vi "processPubDataSubscribe.vi"(8 "error in (no error)":errorcluster, 11 "MiddlewareSALThisComponent in":refnum<class "MiddlewareSALThisComponent.lvclass">) -> (0 "error out":errorcluster, 3 "MiddlewareSALThisComponent out":refnum<class "MiddlewareSALThisComponent.lvclass">)   [LabVIEW 2016, in "MiddlewareSALThisComponent.lvclass"]
uses:
  MiddlewareSALThisComponent.lvclass
  home/harini/tcs/ts_sedspectrometer/ComponentTemplateCore/ComponentModel/ComponentModel/Middleware/Middleware.lvclass
  ComponentTemplateCore/ComponentModel/ComponentModel/Middleware/Middleware.lvclass/Middleware.ctl
  ComponentTemplateCore/ComponentModel/ComponentModel/MiddlewareProcessEvent/MiddlewareProcessEvent.lvclass/MiddlewareProcessEvent.ctl
  PubSubDataEvent/PubSubDataEvent.lvclass/PubSubDataEvent.ctl
  ComponentTemplateCore/ComponentModel/ComponentModel/Middleware/Middleware.lvclass
  ComponentTemplateCore/ComponentModel/ComponentModel/MiddlewareProcessEvent/MiddlewareProcessEvent.lvclass
  PubSubDataEvent/PubSubDataEvent.lvclass
  ProgrammaticInitialization/ProgrammaticInitialization.lvclass
  ts_sallv_sedspectrometer/SALLV_calibrationSpectrometer.lvlib
panel:
  out "stopIsTrue":bool
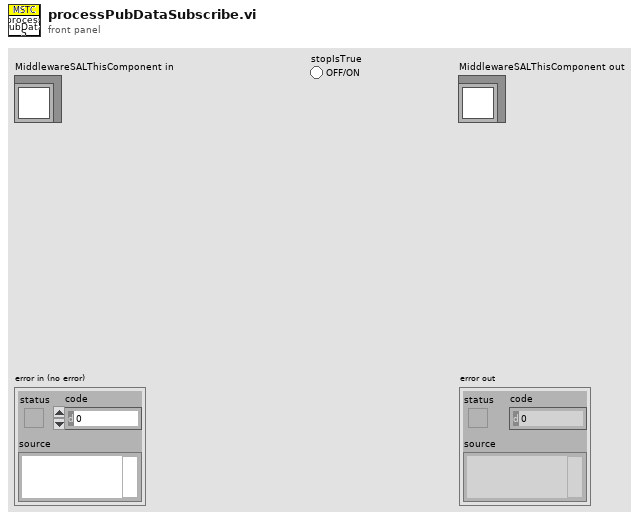
[diagram p1: front panel]
types:
  T1 = typedef "MiddlewareProcessEvents.ctl" = cluster{"disconnect":refnum<user-event>, "error":refnum<user-event>}
  T2 = cluster{"Event Registration Refnum":refnum<event-registration>, "Event Registration Refnum":refnum<event-registration>}
  T3 = typedef "TypedefsDataEvents.lvlib/PubDataEvents.ctl" = cluster{"AppliedSettingsMatchStart":refnum<user-event>, "SettingVersions":refnum<user-event>, "SummaryState":refnum<user-event>, "RejectedCommand":refnum<user-event>, "DetailedState":refnum<user-event>, "ErrorCode":refnum<user-event>, "Heartbeat":refnum<user-event>, "LoopTime_ms":refnum<user-event>, "LoopTimeOutOfRange":refnum<user-event>, "Timestamp":refnum<user-event>, "TimeOut":refnum<user-event>, "MeasuredSpectrum":refnum<user-event>}
  T4 = typedef "SALLV_calibrationSpectrometer.lvlib/logevent_DetailedState.ctl" = cluster{"detailedState":enum16{"", "DisabledState", "EnabledState", "FaultState", "OfflineState", "StandbyState"}, "priority":i32}
  T5 = typedef "SALLV_calibrationSpectrometer.lvlib/logevent_ErrorCode.ctl" = cluster{"errorCode":i32, "priority":i32}
  T6 = typedef "SALLV_calibrationSpectrometer.lvlib/logevent_Heartbeat.ctl" = cluster{"heartbeat":bool, "priority":i32}
  T7 = typedef "SALLV_calibrationSpectrometer.lvlib/LoopTime_ms.ctl" = cluster{"loopTime_ms":dbl}
  T8 = typedef "SALLV_calibrationSpectrometer.lvlib/logevent_LoopTimeOutOfRange.ctl" = cluster{"loopTimeOutOfRange":bool, "priority":i32}
  T9 = typedef "SALLV_calibrationSpectrometer.lvlib/logevent_RejectedCommand.ctl" = cluster{"commandValue":u16, "detailedState":enum16{"", "DisabledState", "EnabledState", "FaultState", "OfflineState", "StandbyState"}, "timestamp":dbl, "priority":i32}
  T10 = typedef "SALLV_calibrationSpectrometer.lvlib/logevent_SummaryState.ctl" = cluster{"summaryState":enum16{"", "DisabledState", "EnabledState", "FaultState", "OfflineState", "StandbyState"}, "priority":i32}
  T11 = typedef "SALLV_calibrationSpectrometer.lvlib/Timestamp.ctl" = cluster{"timestamp":dbl}
  T12 = typedef "SALLV_calibrationSpectrometer.lvlib/logevent_SettingVersions.ctl" = cluster{"recommendedSettingsVersion":string, "recommendedSettingsLabels":string, "priority":i32}
  T13 = typedef "SALLV_calibrationSpectrometer.lvlib/logevent_MeasuredSpectrum.ctl" = cluster{"spectId":u16, "wavelength[2048]":dbl[], "intensity[2048]":dbl[], "imageName":string, "priority":i32}
  T14 = typedef "SALLV_calibrationSpectrometer.lvlib/logevent_TimeOut.ctl" = cluster{"Timeout":bool, "priority":i32}
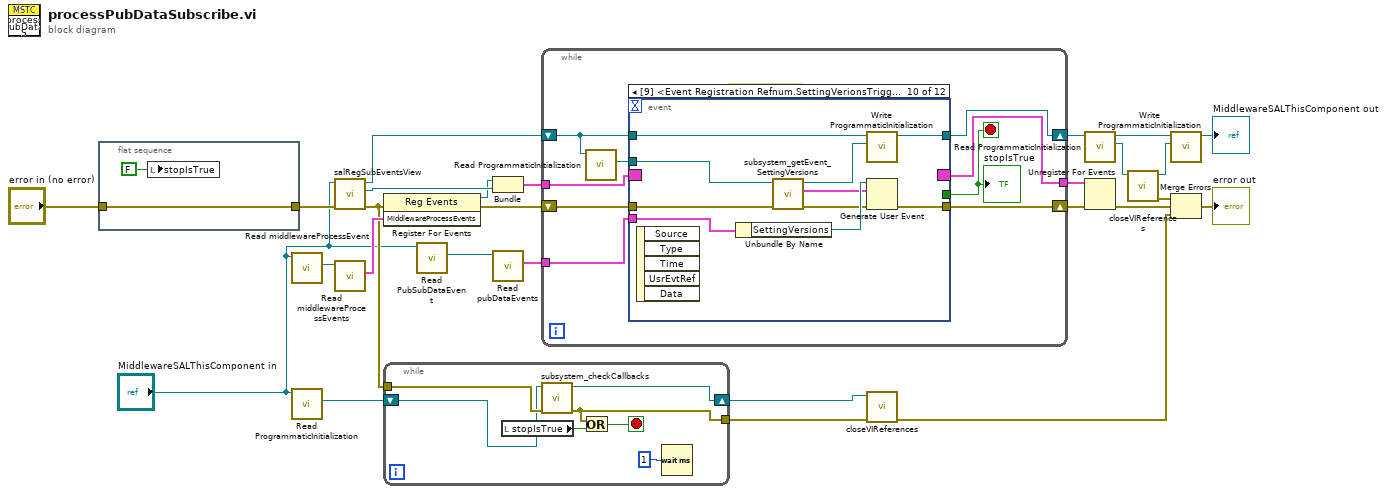
[diagram p0: block diagram]
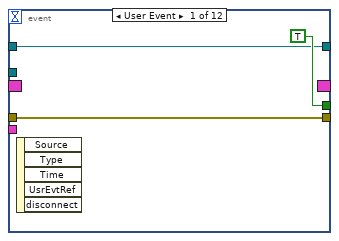
[diagram p2: hidden frame]
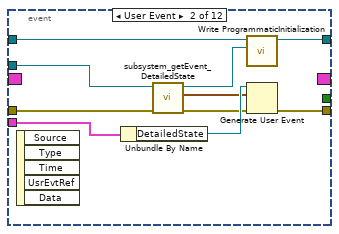
[diagram p3: hidden frame]
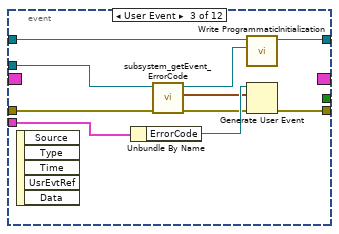
[diagram p4: hidden frame]
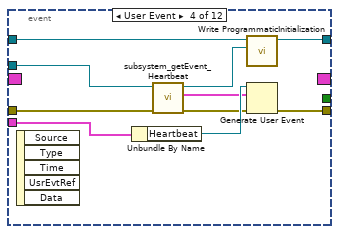
[diagram p5: hidden frame]
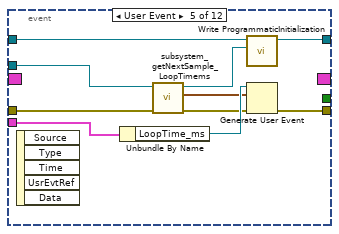
[diagram p6: hidden frame]
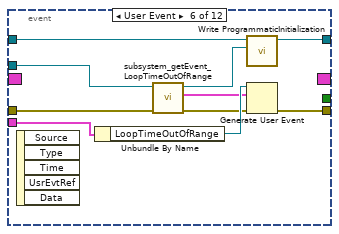
[diagram p7: hidden frame]
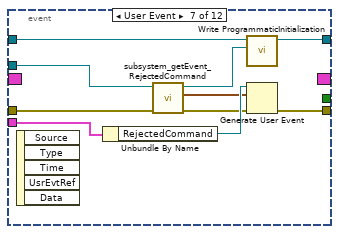
[diagram p8: hidden frame]
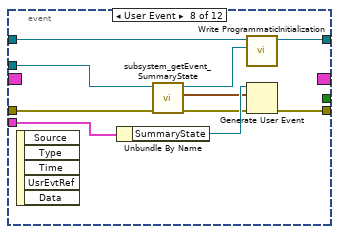
[diagram p9: hidden frame]
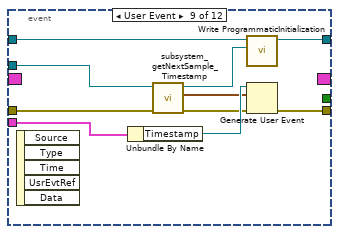
[diagram p10: hidden frame]
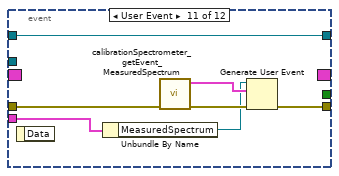
[diagram p11: hidden frame]
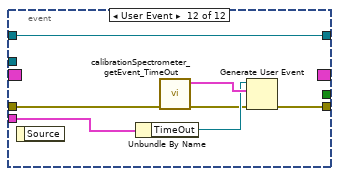
[diagram p12: hidden frame]
diagram:
  n1 = flat-sequence {
    tunnel: "error in (no error)" -> [w29]
    tunnel: [w29] -> w21
    frame #0 {
      n2 = local write "stopIsTrue"(FALSE ("stopIsTrue")) -> ()
    }
  }
  n3 = call "Read middlewareProcessEvent.vi"("Middleware in"="MiddlewareSALThisComponent in") -> ("middlewareProcessEvent"=w26:refnum<class "MiddlewareProcessEvent.lvclass">)  [unwired: 9 in, 1 out]
  n4 = call-dynamic "Read ProgrammaticInitialization.vi"("MiddlewareSALThisComponent in"="MiddlewareSALThisComponent in") -> ("ProgrammaticInitialization"=w10:refnum<class "ProgrammaticInitialization.lvclass">)  [unwired: 8 in, 2 out]
  n5 = call "salRegSubEventsView.vi"("error in (no error)"=w21, "MiddlewareSALThisComponent in"="MiddlewareSALThisComponent in") -> ("error out"=w15:errorcluster, "Event Registration Refnum"=w18:refnum<event-registration>, "MiddlewareSALThisComponent out"=w23:refnum<class "MiddlewareSALThisComponent.lvclass">)  [unwired: 7 in]
  n6 = call "Read middlewareProcessEvents.vi"("MiddlewareProcessEvent in"=w26) -> ("MiddlewareProcessEvents"=w16:T1)  [unwired: 9 in, 1 out]
  n7 = register-events(error in=w15, w16) -> (reference out=w17:refnum<event-registration>, error out=w14:errorcluster)  [unwired: 1 in]
  n8 = while {
    tunnel: [w33] -> w8
    tunnel: w15 -> [w32]
    shift-right: [w30] -> w9
    shift-left: w10 -> [w31]
    stop <- w35 stop-if-true
    n9 = local read "stopIsTrue"() -> (w34:bool)
    n10 = call "subsystem_checkCallbacks.vi"("error in (no error)"=w32, "ProgrammaticInitialization in"=w31) -> ("error out"=w33:errorcluster, "ProgrammaticInitialization out"=w30:refnum<class "ProgrammaticInitialization.lvclass">)  [unwired: 8 in]
    n11 = Or(x=w33, y=w34) -> (x .or. y?=w35:bool)
    n12 = Wait (ms)(milliseconds to wait=u32 1) -> ()  [unwired: 1 out]
  }
  n13 = call-dynamic "Read PubSubDataEvent.vi"("MiddlewareSALThisComponent in"="MiddlewareSALThisComponent in") -> ("PubSubDataEvent.lvclass"=w12:refnum<class "PubSubDataEvent.lvclass">)  [unwired: 8 in, 2 out]
  n14 = Bundle("Event Registration Refnum"=w17, "Event Registration Refnum"=w18) -> (w19:T2)  [unwired: 1 in]
  n15 = call "Read pubDataEvents.vi"("PubSubDataEvent in"=w12) -> ("pubDataEvents"=w13:T3)  [unwired: 9 in, 1 out]
  n16 = while {
    tunnel: w19 -> [w41]
    tunnel: [w45] -> w20
    shift-right: [w44] -> w6
    shift-left: w23 -> [w38]
    shift-right: [w42] -> w27
    shift-left: w14 -> [w39]
    tunnel: w13 -> [w40]
    stop <- w43 stop-if-true
    # "Fix timestamps"
    n17 = call-dynamic "Read ProgrammaticInitialization.vi"("MiddlewareSALThisComponent in"=w38) -> ("ProgrammaticInitialization"=w37:refnum<class "ProgrammaticInitialization.lvclass">)  [unwired: 8 in, 2 out]
    n18 = event shown="[9] <Event Registration Refnum.SettingVerionsTriggered>: User Event" {
      selector: w41 -> [_ _ _ _ _ _ _ _ _ _ _ _]
      dyn-events: [_ _ _ _ _ _ _ _ _ _ _ _] -> w45
      timeout: _ -> [_ _ _ _ _ _ _ _ _ _ _ _]
      tunnel: [TRUE ("stopIsTrue") _ _ _ _ _ _ _ _ _ _ _] -> w43
      tunnel: w38 -> [w47 w52 w62 w72 w82 w92 w102 w112 w122 w131 w139 w146]
      tunnel: [w47 w51 w61 w71 w81 w91 w101 w111 w121 w130 w139 w146] -> w44
      tunnel: w39 -> [w46 w54 w64 w74 w84 w94 w104 w114 w124 w133 w140 w147]
      tunnel: [w46 w57 w67 w77 w87 w97 w107 w117 w127 w136 w141 w149] -> w42
      tunnel: w40 -> [_ w58 w68 w78 w88 w98 w108 w118 w128 w137 w143 w151]
      tunnel: w37 -> [_ w53 w63 w73 w83 w93 w103 w113 w123 w132 _ _]
      event User Event {
        n19 = event-data() -> ()  [unwired: 1 in, 5 out]
      }
      event User Event {
        n20 = event-data() -> ()  [unwired: 1 in, 5 out]
        n21 = Unbundle By Name(w58) -> ("DetailedState"=w56:refnum<user-event>)
        n22 = call "subsystem_getEvent_DetailedState.vi"("error in (no error)"=w54, "ProgrammaticInitialization in"=w53) -> ("error out"=w55:errorcluster, "logevent_DetailedState"=w49:T4, "ProgrammaticInitialization out"=w50:refnum<class "ProgrammaticInitialization.lvclass">)  [unwired: 7 in]
        n23 = call-dynamic "Write ProgrammaticInitialization.vi"("ProgrammaticInitialization.lvclass"=w50, "MiddlewareSALThisComponent in"=w52) -> ("MiddlewareSALThisComponent out"=w51:refnum<class "MiddlewareSALThisComponent.lvclass">)  [unwired: 8 in, 1 out]
        n24 = Generate User Event(user event=w56, event data cluster=w49, error in=w55) -> (error out=w57:errorcluster)  [unwired: 1 in, 1 out]
      }
      event User Event {
        n25 = event-data() -> ()  [unwired: 1 in, 5 out]
        n26 = Unbundle By Name(w68) -> ("ErrorCode"=w66:refnum<user-event>)
        n27 = call "subsystem_getEvent_ErrorCode.vi"("error in (no error)"=w64, "ProgrammaticInitialization in"=w63) -> ("error out"=w65:errorcluster, "logevent_ErrorCode"=w59:T5, "ProgrammaticInitialization out"=w60:refnum<class "ProgrammaticInitialization.lvclass">)  [unwired: 7 in]
        n28 = call-dynamic "Write ProgrammaticInitialization.vi"("ProgrammaticInitialization.lvclass"=w60, "MiddlewareSALThisComponent in"=w62) -> ("MiddlewareSALThisComponent out"=w61:refnum<class "MiddlewareSALThisComponent.lvclass">)  [unwired: 8 in, 1 out]
        n29 = Generate User Event(user event=w66, event data cluster=w59, error in=w65) -> (error out=w67:errorcluster)  [unwired: 1 in, 1 out]
      }
      event User Event {
        n30 = event-data() -> ()  [unwired: 1 in, 5 out]
        n31 = Unbundle By Name(w78) -> ("Heartbeat"=w76:refnum<user-event>)
        n32 = call "subsystem_getEvent_Heartbeat.vi"("error in (no error)"=w74, "ProgrammaticInitialization in"=w73) -> ("error out"=w75:errorcluster, "logevent_Heartbeat"=w69:T6, "ProgrammaticInitialization out"=w70:refnum<class "ProgrammaticInitialization.lvclass">)  [unwired: 7 in]
        n33 = call-dynamic "Write ProgrammaticInitialization.vi"("ProgrammaticInitialization.lvclass"=w70, "MiddlewareSALThisComponent in"=w72) -> ("MiddlewareSALThisComponent out"=w71:refnum<class "MiddlewareSALThisComponent.lvclass">)  [unwired: 8 in, 1 out]
        n34 = Generate User Event(user event=w76, event data cluster=w69, error in=w75) -> (error out=w77:errorcluster)  [unwired: 1 in, 1 out]
      }
      event User Event {
        n35 = event-data() -> ()  [unwired: 1 in, 5 out]
        n36 = Unbundle By Name(w88) -> ("LoopTime_ms"=w86:refnum<user-event>)
        n37 = call "subsystem_getNextSample_LoopTimems.vi"("error in (no error)"=w84, "ProgrammaticInitialization in"=w83) -> ("error out"=w85:errorcluster, "LoopTime_ms out"=w79:T7, "ProgrammaticInitialization out"=w80:refnum<class "ProgrammaticInitialization.lvclass">)  [unwired: 7 in]
        n38 = call-dynamic "Write ProgrammaticInitialization.vi"("ProgrammaticInitialization.lvclass"=w80, "MiddlewareSALThisComponent in"=w82) -> ("MiddlewareSALThisComponent out"=w81:refnum<class "MiddlewareSALThisComponent.lvclass">)  [unwired: 8 in, 1 out]
        n39 = Generate User Event(user event=w86, event data cluster=w79, error in=w85) -> (error out=w87:errorcluster)  [unwired: 1 in, 1 out]
      }
      event User Event {
        n40 = event-data() -> ()  [unwired: 1 in, 5 out]
        n41 = Unbundle By Name(w98) -> ("LoopTimeOutOfRange"=w96:refnum<user-event>)
        n42 = call "subsystem_getEvent_LoopTimeOutOfRange.vi"("error in (no error)"=w94, "ProgrammaticInitialization in"=w93) -> ("error out"=w95:errorcluster, "logevent_LoopTimeOutOfRange"=w89:T8, "ProgrammaticInitialization out"=w90:refnum<class "ProgrammaticInitialization.lvclass">)  [unwired: 7 in]
        n43 = call-dynamic "Write ProgrammaticInitialization.vi"("ProgrammaticInitialization.lvclass"=w90, "MiddlewareSALThisComponent in"=w92) -> ("MiddlewareSALThisComponent out"=w91:refnum<class "MiddlewareSALThisComponent.lvclass">)  [unwired: 8 in, 1 out]
        n44 = Generate User Event(user event=w96, event data cluster=w89, error in=w95) -> (error out=w97:errorcluster)  [unwired: 1 in, 1 out]
      }
      event User Event {
        n45 = event-data() -> ()  [unwired: 1 in, 5 out]
        n46 = Unbundle By Name(w108) -> ("RejectedCommand"=w106:refnum<user-event>)
        n47 = call "subsystem_getEvent_RejectedCommand.vi"("error in (no error)"=w104, "ProgrammaticInitialization in"=w103) -> ("error out"=w105:errorcluster, "logevent_RejectedCommand"=w99:T9, "ProgrammaticInitialization out"=w100:refnum<class "ProgrammaticInitialization.lvclass">)  [unwired: 7 in]
        n48 = call-dynamic "Write ProgrammaticInitialization.vi"("ProgrammaticInitialization.lvclass"=w100, "MiddlewareSALThisComponent in"=w102) -> ("MiddlewareSALThisComponent out"=w101:refnum<class "MiddlewareSALThisComponent.lvclass">)  [unwired: 8 in, 1 out]
        n49 = Generate User Event(user event=w106, event data cluster=w99, error in=w105) -> (error out=w107:errorcluster)  [unwired: 1 in, 1 out]
      }
      event User Event {
        n50 = event-data() -> ()  [unwired: 1 in, 5 out]
        n51 = Unbundle By Name(w118) -> ("SummaryState"=w116:refnum<user-event>)
        n52 = call "subsystem_getEvent_SummaryState.vi"("error in (no error)"=w114, "ProgrammaticInitialization in"=w113) -> ("error out"=w115:errorcluster, "logevent_SummaryState"=w109:T10, "ProgrammaticInitialization out"=w110:refnum<class "ProgrammaticInitialization.lvclass">)  [unwired: 7 in]
        n53 = call-dynamic "Write ProgrammaticInitialization.vi"("ProgrammaticInitialization.lvclass"=w110, "MiddlewareSALThisComponent in"=w112) -> ("MiddlewareSALThisComponent out"=w111:refnum<class "MiddlewareSALThisComponent.lvclass">)  [unwired: 8 in, 1 out]
        n54 = Generate User Event(user event=w116, event data cluster=w109, error in=w115) -> (error out=w117:errorcluster)  [unwired: 1 in, 1 out]
      }
      event User Event {
        n55 = event-data() -> ()  [unwired: 1 in, 5 out]
        n56 = Unbundle By Name(w128) -> ("Timestamp"=w126:refnum<user-event>)
        n57 = call "subsystem_getNextSample_Timestamp.vi"("error in (no error)"=w124, "ProgrammaticInitialization in"=w123) -> ("error out"=w125:errorcluster, "Timestamp out"=w119:T11, "ProgrammaticInitialization out"=w120:refnum<class "ProgrammaticInitialization.lvclass">)  [unwired: 7 in]
        n58 = call-dynamic "Write ProgrammaticInitialization.vi"("ProgrammaticInitialization.lvclass"=w120, "MiddlewareSALThisComponent in"=w122) -> ("MiddlewareSALThisComponent out"=w121:refnum<class "MiddlewareSALThisComponent.lvclass">)  [unwired: 8 in, 1 out]
        n59 = Generate User Event(user event=w126, event data cluster=w119, error in=w125) -> (error out=w127:errorcluster)  [unwired: 1 in, 1 out]
      }
      event User Event {
        n60 = event-data() -> ()  [unwired: 1 in, 5 out]
        n61 = Unbundle By Name(w137) -> ("SettingVersions"=w138:refnum<user-event>)
        n62 = call "subsystem_getEvent_SettingVersions.vi"("error in (no error)"=w133, "ProgrammaticInitialization in"=w132) -> ("error out"=w134:errorcluster, "logevent_SettingVersions"=w135:T12, "ProgrammaticInitialization out"=w129:refnum<class "ProgrammaticInitialization.lvclass">)  [unwired: 7 in]
        n63 = call-dynamic "Write ProgrammaticInitialization.vi"("ProgrammaticInitialization.lvclass"=w129, "MiddlewareSALThisComponent in"=w131) -> ("MiddlewareSALThisComponent out"=w130:refnum<class "MiddlewareSALThisComponent.lvclass">)  [unwired: 8 in, 1 out]
        n64 = Generate User Event(user event=w138, event data cluster=w135, error in=w134) -> (error out=w136:errorcluster)  [unwired: 1 in, 1 out]
      }
      event User Event {
        n65 = event-data() -> ()  [unwired: 1 in, 1 out]
        n66 = Unbundle By Name(w143) -> ("MeasuredSpectrum"=w142:refnum<user-event>)
        n67 = call "calibrationSpectrometer_getEvent_MeasuredSpectrum.vi"("error in (no error)"=w140) -> ("error out"=w145:errorcluster, "logevent_MeasuredSpectrum_Ctl out"=w144:T13)  [unwired: 8 in, 1 out]
        n68 = Generate User Event(user event=w142, event data cluster=w144, error in=w145) -> (error out=w141:errorcluster)  [unwired: 1 in, 1 out]
      }
      event User Event {
        n69 = event-data() -> ()  [unwired: 1 in, 1 out]
        n70 = Unbundle By Name(w151) -> ("TimeOut"=w150:refnum<user-event>)
        n71 = call "calibrationSpectrometer_getEvent_TimeOut.vi"("error in (no error)"=w147) -> ("error out"=w148:errorcluster, "logevent_TimeOut_Ctl out"=w152:T14)  [unwired: 8 in, 1 out]
        n72 = Generate User Event(user event=w150, event data cluster=w152, error in=w148) -> (error out=w149:errorcluster)  [unwired: 1 in, 1 out]
      }
    }
    "stopIsTrue" <- w43
  }
  n73 = call "closeVIReferences.vi"("error in (no error)"=w8, "ProgrammaticInitialization in"=w9) -> ("error out"=w7:errorcluster)  [unwired: 8 in, 1 out]
  n74 = call-dynamic "Read ProgrammaticInitialization.vi"("MiddlewareSALThisComponent in"=w6) -> ("ProgrammaticInitialization"=w5:refnum<class "ProgrammaticInitialization.lvclass">, "MiddlewareSALThisComponent out"=w4:refnum<class "MiddlewareSALThisComponent.lvclass">)  [unwired: 8 in, 1 out]
  n75 = Unregister For Events(event registration refnum=w20, error in=w27) -> (error out=w24:errorcluster)
  n76 = call "closeVIReferences.vi"("ProgrammaticInitialization in"=w5) -> ("error out"=w1:errorcluster, "ProgrammaticInitialization out"=w3:refnum<class "ProgrammaticInitialization.lvclass">)  [unwired: 9 in]
  n77 = call-dynamic "Write ProgrammaticInitialization.vi"("ProgrammaticInitialization.lvclass"=w3, "MiddlewareSALThisComponent in"=w4) -> ("MiddlewareSALThisComponent out"=→"MiddlewareSALThisComponent out":refnum<class "MiddlewareSALThisComponent.lvclass">)  [unwired: 8 in, 1 out]
  n78 = Merge Errors(w1, w24, w7) -> (→"error out":errorcluster)
